vi "LV algorithm bias.vi"(0 "data":dbl[](array[numeric]), 1 "B0":dbl[](array[numeric])=[1.0, 1.0, 1.0]) -> (2 "B new":dbl[](array[numeric]), 3 "Error B":dbl, 4 "Interation Error Graph":dbl[](graph), 5 "data processed":cluster{dbl[]}[](graph))   [LabVIEW 2021, in "IMU Processing.lvlib"]
uses:
  IMU Processing.lvlib
  <vilib>/Analysis/7linalg.llb/Real Transpose Matrix.vi
  <vilib>/Analysis/baseanly.llb/Real A x B.vi
  <vilib>/Analysis/baseanly.llb/A x Vector.vi
  <vilib>/Analysis/Matrix/Numeric/Conversions/Matrix To Array - RM.vi
  <vilib>/Analysis/7linalg.llb/Create Special Real Matrix.vi
  <vilib>/Analysis/NI_AALBase.lvlib
  <vilib>/Analysis/NI_AALPro.lvlib
  <vilib>/Analysis/Matrix/NI_Matrix.lvlib
panel:
  out "i":i32
  in  "y0":dbl=-10.0
  out "y":dbl=1.0
  out "Error B old":dbl
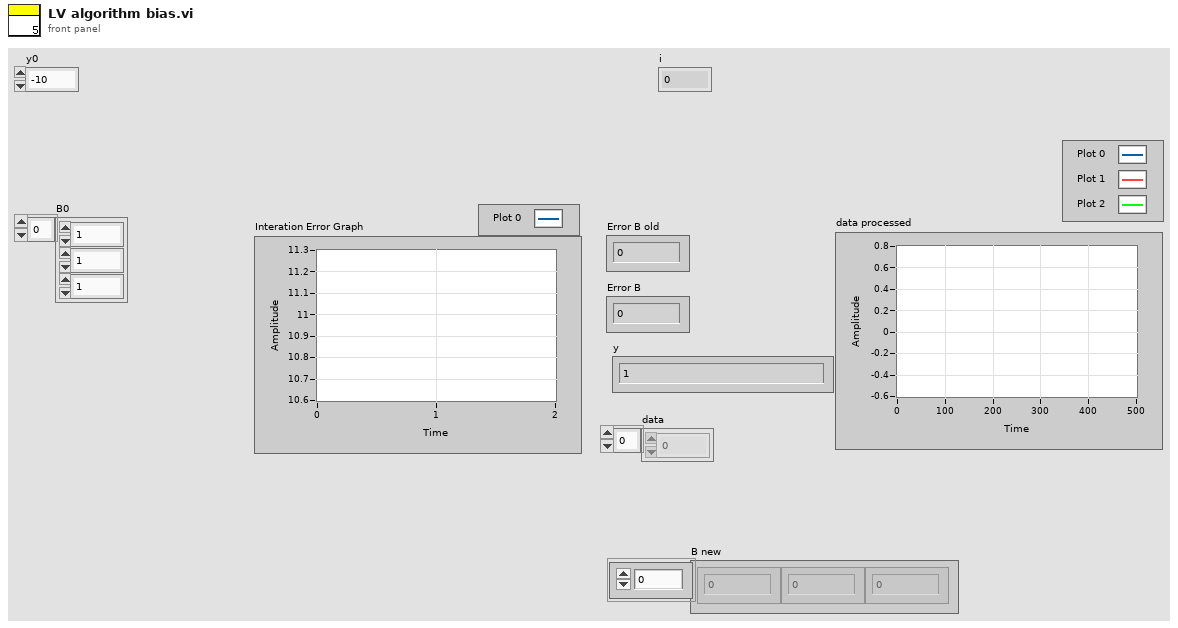
[diagram p1: front panel]
types:
  T1 = typedef "NI_Matrix.lvlib/RealMatrix.ctl" = dbl[][]
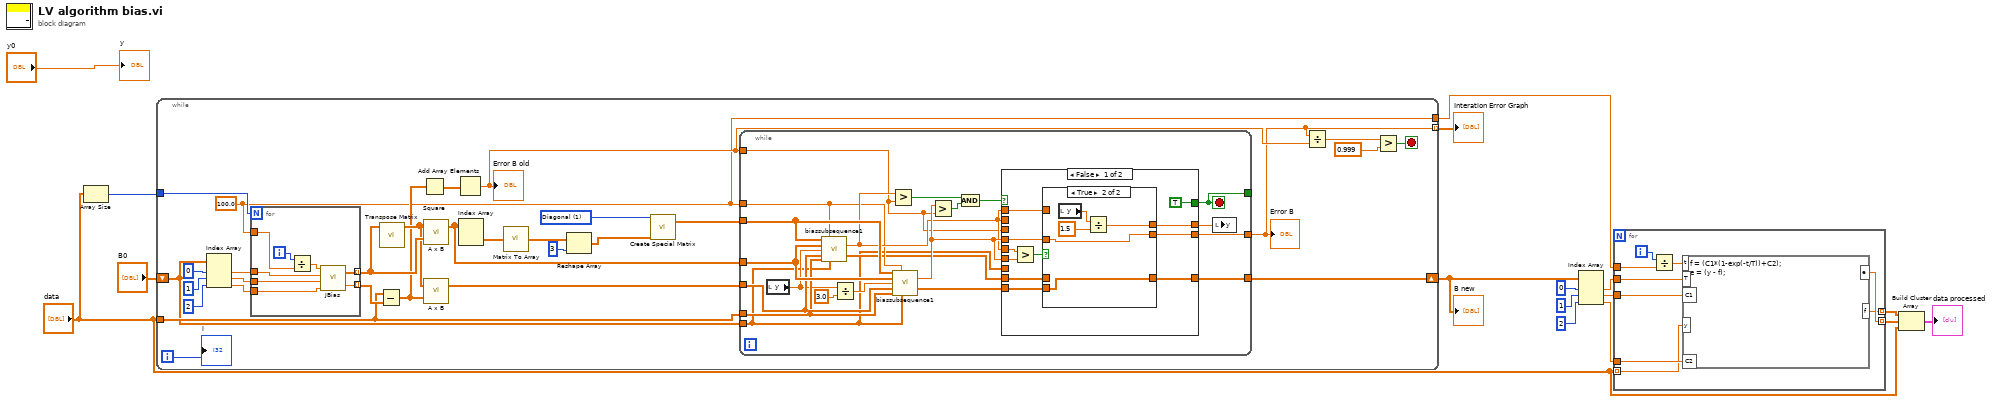
[diagram p0: block diagram]
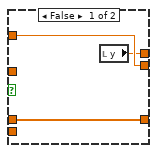
[diagram p2: hidden frame]
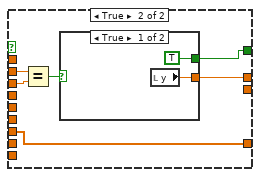
[diagram p3: hidden frame]
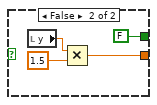
[diagram p4: hidden frame]
diagram:
  n1 = Array Size(array="data") -> (size(s)=w16:i32)
  n2 = while {
    tunnel: [w21] -> w14 mode=indexing
    tunnel: w16 -> [w23]
    tunnel: "data" -> [w22]
    shift-right: [w18] -> w10
    shift-left: "B0" -> [w20]
    tunnel: [w19] -> w6
    i -> [w17]
    stop <- w24 stop-if-true
    w19 = 100.0 ("frequency")
    w44 = 1 items=["Identity", "Diagonal", "Toeplitz", "Vandermonde", "Companion", "Hankel", "Hadamard", "Wilkinson", "Hilbert", "Inverse Hilbert", "Rosser", "Pascal"] ("matrix type")
    n3 = Index Array(array=w20, index #1=0 ("index"), index #2=1 ("index"), index #3=2 ("index")) -> (element #1=w30:dbl, element #2=w29:dbl, element #3=w28:dbl)
    n4 = for {
      N: w23 -> [_]
      tunnel: w30 -> [w104]
      tunnel: w29 -> [w103]
      tunnel: w28 -> [w102]
      tunnel: [w101] -> w46 mode=indexing
      tunnel: [w100] -> w38 mode=indexing
      tunnel: w19 -> [w99]
      i -> [w106]
      n5 = Divide(x=w106, y=w99) -> (x/y=w105:dbl)
      n6 = call "JBias.vi"("C2"=w102, "C1"=w103, "T"=w104, "t"=w105) -> ("f(t)"=w100:dbl, "Jbias"=w101:dbl[])
    }
    n7 = Subtract(x=w22, y=w38) -> (x-y=w35:dbl[])
    n8 = call-poly <vilib>:"Transpose Matrix.vi"("Input Matrix"=w46) -> ("Matrix Transpose"=w37:T1)  [unwired: 9 in, 1 out]
    n9 = Square(x=w35) -> (x^2=w34:dbl[])
    n10 = call-poly <vilib>:"A x B.vi"("B"=w46, "A"=w37) -> ("A x B"=w45:T1)  [unwired: 1 out]
    n11 = call-poly <vilib>:"A x B.vi"("Vector"=w35, "A"=w37) -> ("A x Vector"=w36:dbl[])  [unwired: 1 out]
    n12 = Add Array Elements(numeric array=w34) -> (sum=w25:dbl)
    "Error B old" <- w25
    n13 = Index Array(array=w45) -> (element=w42:T1)  [unwired: 2 in]
    n14 = call-poly <vilib>:"Matrix To Array.vi"("Real Matrix"=w42) -> ("Real 2D Array"=w41:dbl[][])
    n15 = Reshape Array(w41, 3 ("dimension size")) -> (w40:dbl[])
    n16 = call-poly <vilib>:"Create Special Matrix.vi"("matrix type"=w44, "Input Vector1"=w40) -> ("Special Matrix"=w43:T1)  [unwired: 3 in, 1 out]
    n17 = while {
      tunnel: w45 -> [w66]
      tunnel: w43 -> [w67]
      tunnel: w36 -> [w65]
      tunnel: w20 -> [w47]
      tunnel: w25 -> [w56]
      tunnel: [w59] -> w21
      tunnel: [w55] -> _
      tunnel: w22 -> [w54]
      tunnel: w19 -> [w51]
      tunnel: [w50] -> w18
      stop <- w55 stop-if-true
      n18 = local read "y"() -> (w52:dbl)
      n19 = call "biassubsequence1.vi"("diag(J'J)"=w67, "frequency"=w51, "J'J"=w66, "delta"=w52, "J'(y-f(t))"=w65, "y"=w54, "B old"=w47) -> ("error"=w57:dbl, "B new"=w49:dbl[])  [unwired: 7 in]
      n20 = Divide(x=w52, y=3.0) -> (x/y=w63:dbl)
      n21 = Greater?(x=w57, y=w56) -> (0:w62:bool)
      n22 = call "biassubsequence1.vi"("diag(J'J)"=w67, "frequency"=w51, "J'J"=w66, "delta"=w63, "J'(y-f(t))"=w65, "y"=w54, "B old"=w47) -> ("error"=w58:dbl, "B new"=w48:dbl[])  [unwired: 7 in]
      n23 = Greater?(x=w58, y=w56) -> (0:w61:bool)
      n24 = And(x=w62, y=w61) -> (x .and. y?=w60:bool)
      n25 = case shown="False" w60 {
        tunnel: [TRUE w88] -> w55
        tunnel: [w74 w92] -> w53
        tunnel: w57 -> [w76 _]
        tunnel: w58 -> [w77 _]
        tunnel: [w73 _] -> w59
        tunnel: w58 -> [w72 _]
        tunnel: w57 -> [w71 _]
        tunnel: w57 -> [_ w90]
        tunnel: w56 -> [_ w91]
        tunnel: [w70 w87] -> w50
        tunnel: w49 -> [w69 _]
        tunnel: w48 -> [w68 _]
        tunnel: w47 -> [_ w87]
        frame False {
          n26 = Greater?(x=w76, y=w77) -> (0:w75:bool)
          n27 = case shown="True" w75 {
            tunnel: [w80 w85] -> w74
            tunnel: [w81 w84] -> w73
            tunnel: w72 -> [_ w84]
            tunnel: w71 -> [w81 _]
            tunnel: [w79 w82] -> w70
            tunnel: w69 -> [w79 _]
            tunnel: w68 -> [_ w82]
            frame False {
              n28 = local read "y"() -> (w80:dbl)
            }
            frame True {
              n29 = local read "y"() -> (w83:dbl)
              n30 = Divide(x=w83, y=1.5) -> (x/y=w85:dbl)
            }
          }
        }
        frame True {
          n31 = Equal?(x=w90, y=w91) -> (x = y?=w89:bool)
          n32 = case shown="True" w89 {
            tunnel: [w93 w97] -> w92
            tunnel: [TRUE FALSE] -> w88
            frame True {
              n33 = local read "y"() -> (w93:dbl)
            }
            frame False {
              n34 = local read "y"() -> (w95:dbl)
              n35 = Multiply(x=w95, y=1.5) -> (x*y=w97:dbl)
            }
          }
        }
      }
      n36 = local write "y"(w53) -> ()
    }
    "Error B" <- w21
    n37 = Divide(x=w21, y=w25) -> (x/y=w27:dbl)
    n38 = Greater?(x=w27, y=0.999) -> (0:w24:bool)
    "i" <- w17
  }
  "Interation Error Graph" <- w14
  "B new" <- w10
  n39 = Index Array(array=w10, index #1=0 ("index"), index #2=1 ("index"), index #3=2 ("index")) -> (element #1=w9:dbl, element #2=w8:dbl, element #3=w7:dbl)
  n40 = for {
    tunnel: "data" -> [w110] mode=indexing
    tunnel: w9 -> [w113]
    tunnel: w8 -> [w112]
    tunnel: w7 -> [w111]
    tunnel: [w109] -> w4 mode=indexing
    tunnel: w6 -> [w108]
    tunnel: [w107] -> w2 mode=indexing
    i -> [w115]
    n41 = Divide(x=w115, y=w108) -> (x/y=w114:dbl)
    n42 = formula code="f = (C1*(1-exp(-t/T))+C2);\ne = (y - f);"("t"=w114, "T"=w113, "C1"=w112, "C2"=w111, "y"=w110) -> ("e"=w109:dbl, "f"=w107:dbl)
  }
  n43 = Build Cluster Array(w2, w4, "data") -> (→"data processed":cluster{"data":dbl[]}[])
  "y" <- "y0"
